vi "FG COP RBT VelocityState.vi"(1 "FG Action (Read)":T3, 2 "RBT VelocityState in":T1) -> (0 "RBT VelocityState out":T1)   [LabVIEW 2011]
uses:
  cRIO/Functional Global Variables/Actions for FG's.ctl
  Support Files/VelocityState.ctl
  Support Files/TimeRec.ctl
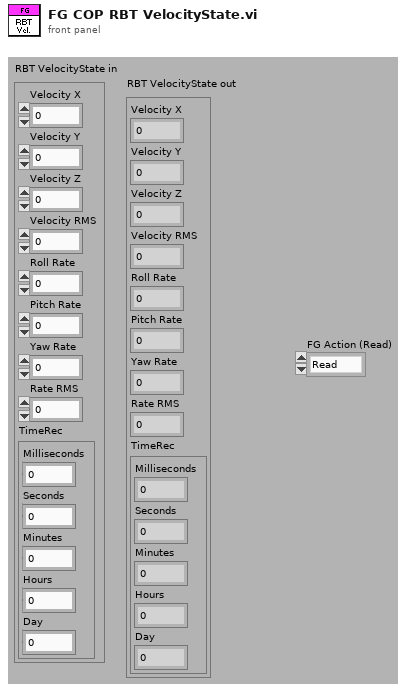
[diagram p1: front panel]
types:
  T1 = typedef "VelocityState.ctl" = cluster{"Velocity X":dbl, "Velocity Y":dbl, "Velocity Z":dbl, "Velocity RMS":dbl, "Roll Rate":dbl, "Pitch Rate":dbl, "Yaw Rate":dbl, "Rate RMS":dbl, "TimeRec":T2}
  T2 = typedef "TimeRec.ctl" = cluster{"Milliseconds":u32, "Seconds":u32, "Minutes":u32, "Hours":u32, "Day":u32}
  T3 = typedef "Actions for FG's.ctl" = enum16{"Read", "Write"}
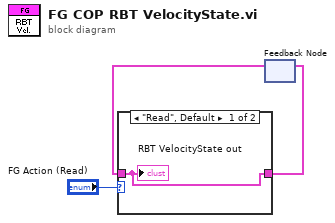
[diagram p0: block diagram]
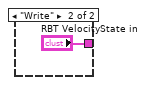
[diagram p2: hidden frame]
diagram:
  n1 = feedback #1() -> (w1:T1)  [unwired: 1 in]
  n2 = case shown="\"Read\", Default" "FG Action (Read)" {
    tunnel: [w4 "RBT VelocityState in"] -> w2
    tunnel: w1 -> [w4 _]
    frame "Read", Default {
      "RBT VelocityState out" <- w4
    }
    frame "Write" {
    }
  }
  n3 = feedback-in #1(w2) -> ()
